vi "Copy Value.vi"(10 "From":refnum<class "Type.lvclass">, 11 "Double in":refnum<class "Double.lvclass">) -> (2 "error out":errorcluster, 3 "Double out":refnum<class "Double.lvclass">)   [LabVIEW 2020, in "Conditu2.lvlib" / "Columns.lvlib" / "Double.lvclass"]
uses:
  Double.lvclass
  Type/Type.lvclass
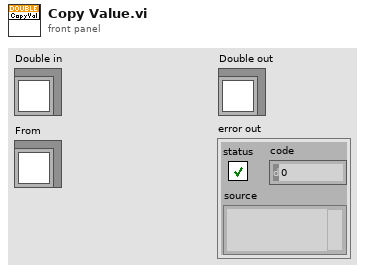
[diagram p1: front panel]
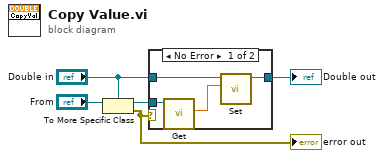
[diagram p0: block diagram]
diagram:
  n1 = To More Specific Class(target class="Double in", reference="From") -> (specific class reference=w5:refnum<class "Double.lvclass">, error out=w1:errorcluster)  [unwired: 1 in]
  "error out" <- w1
  n2 = case shown="No Error" w1 {
    tunnel: w5 -> [w9 _]
    tunnel: "Double in" -> [w7 w10]
    tunnel: [w6 w10] -> w4
    frame No Error {
      n3 = call "Get.vi"("Double in"=w9) -> ("Value"=w8:dbl)  [unwired: 10 in]
      n4 = call "Set.vi"("Value"=w8, "Double in"=w7) -> ("Double out"=w6:refnum<class "Double.lvclass">)  [unwired: 9 in]
    }
    frame Error {
    }
  }
  "Double out" <- w4
